vi "test_CalculateSpecificationBuildOrder_SampleProjectWithExternalDep.vi"() -> (3 "Pass?":bool)   [LabVIEW 2019, in "Tests.SolutionBuilder.lvlib"]
uses:
  Tests.SolutionBuilder.lvlib
  SolutionBuilder/SolutionBuilder.lvclass
  SolutionBuilder/ProjectItem/ProjectItem.lvclass
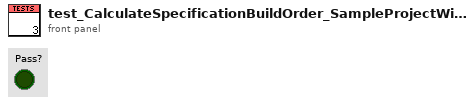
[diagram p1: front panel]
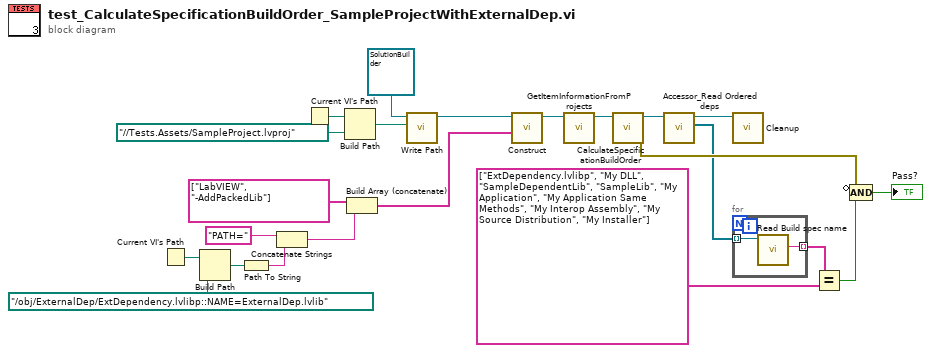
[diagram p0: block diagram]
diagram:
  n1 = Current VI's Path() -> (path=w6:path)
  n2 = Build Path(base path=w6, name or relative path=path "../obj/ExternalDep/ExtDependency.lvlibp::NAME=ExternalDep.lvlib" ("Path")) -> (appended path=w7:path)
  n3 = Path To String(path=w7) -> (string=w4:string)
  n4 = Concatenate Strings("PATH=" ("string"), w4) -> (w2:string)
  n5 = Current VI's Path() -> (path=w22:path)
  n6 = Build Path(base path=w22, name or relative path=path "../../Tests.Assets/SampleProject.lvproj" ("Path")) -> (appended path=w20:path)
  n7 = Build Array (concatenate)(string[] ["LabVIEW", "-AddPackedLib"] ("App.Args"), w2) -> (w16:string[])
  n8 = call "Write Path.vi"("Path"=w20, "SolutionBuilder in"=refnum<class "SolutionBuilder.lvclass"> refnum) -> ("SolutionBuilder out"=w19:refnum<class "SolutionBuilder.lvclass">)  [unwired: 9 in]
  n9 = call "Construct.vi"("App.Args"=w16, "SolutionBuilder in"=w19) -> ("SolutionBuilder out"=w15:refnum<class "SolutionBuilder.lvclass">)  [unwired: 8 in, 1 out]
  n10 = call "GetItemInformationFromProjects.vi"("SolutionBuilder in"=w15) -> ("SolutionBuilder out"=w14:refnum<class "SolutionBuilder.lvclass">)  [unwired: 9 in, 1 out]
  n11 = call "CalculateSpecificationBuildOrder.vi"("SolutionBuilder in"=w14) -> ("error out"=w11:errorcluster, "SolutionBuilder out"=w13:refnum<class "SolutionBuilder.lvclass">)  [unwired: 9 in]
  n12 = call "Accessor_Read Ordered deps.vi"("SolutionBuilder in"=w13) -> ("Ordered deps"=w10:refnum<class "ProjectItem.lvclass">[], "SolutionBuilder out"=w12:refnum<class "SolutionBuilder.lvclass">)  [unwired: 8 in, 1 out]
  n13 = call "Cleanup.vi"("SolutionBuilder in"=w12) -> ()  [unwired: 9 in, 2 out]
  n14 = for {
    tunnel: w10 -> [w25] mode=indexing
    tunnel: [w24] -> w9 mode=indexing
    n15 = call "Read Build spec name.vi"("ProjectItem in"=w25) -> ("Build spec name"=w24:string)  [unwired: 9 in, 1 out]
  }
  n16 = Equal?(x=w9, y=string[] ["ExtDependency.lvlibp", "My DLL", "SampleDependentLib", "SampleLib", "My Application", "My Application Same Methods", "My Interop Assembly", "My Source Distribution", "My Installer"] ("Array")) -> (x = y?=w18:bool)
  n17 = Compound Arithmetic op=AND(invert w11, w18) -> (→"Pass?":bool)
